vi "Init.vi"(4 "Base Path":path, 6 "Template":string, 8 "Project:Active Project":refnum<vi>, 9 "Application Instance":refnum<vi>, 10 "Name":string, 11 "Actor Script Strategy in":refnum<class "Actor Script Strategy.lvclass">) -> (3 "Actor Script Strategy out":refnum<class "Actor Script Strategy.lvclass">)   [LabVIEW 2021, in "_Create From Template.lvlib" / "Script Strategy.lvlib" / "Actor Script Strategy.lvclass"]
uses:
  Actor Script Strategy.lvclass
  Actor Script Strategy.lvclass/Actor Script Strategy.ctl
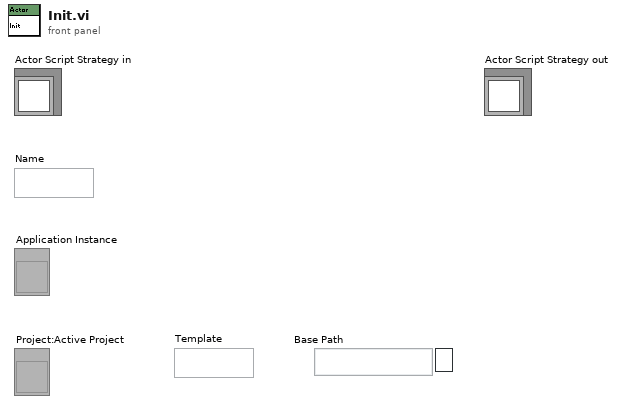
[diagram p1: front panel]
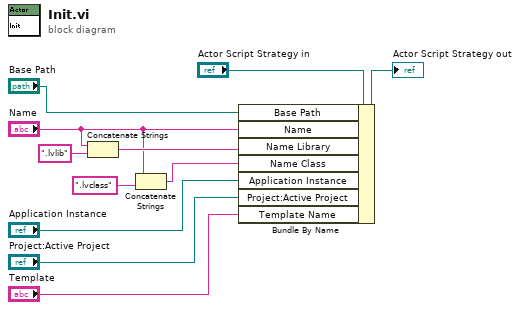
[diagram p0: block diagram]
diagram:
  n1 = Concatenate Strings("Name", ".lvlib" ("string")) -> (w9:string)
  n2 = Concatenate Strings("Name", ".lvclass" ("regular expression")) -> (w7:string)
  n3 = Bundle By Name(cluster="Actor Script Strategy in", "Base Path"="Base Path", "Name"="Name", "Name Library"=w9, "Name Class"=w7, "Application Instance"="Application Instance", "Project:Active Project"="Project:Active Project", "Template Name"="Template") -> (→"Actor Script Strategy out":refnum<class "Actor Script Strategy.lvclass">)
